vi "TestInfo.vi"(4 "Error In":errorcluster, 7 "Command":string) -> (0 "Error Out":errorcluster, 3 "Response":string)   [LabVIEW 2018]
uses:
  MOKO_LabViewLibrary/MokoLowLevel/MokoLowLovelControl/MLLC_Mode.ctl
  data/IZRCSM.ctl
panel:
  in  "Utility name":string="IZRCSM"
  in  "Error Code":i32=5475
  in  "Settings":T2
  in  "Mode":T3=enum."Check"
  # "TestInfo"
  # "Default Settings"
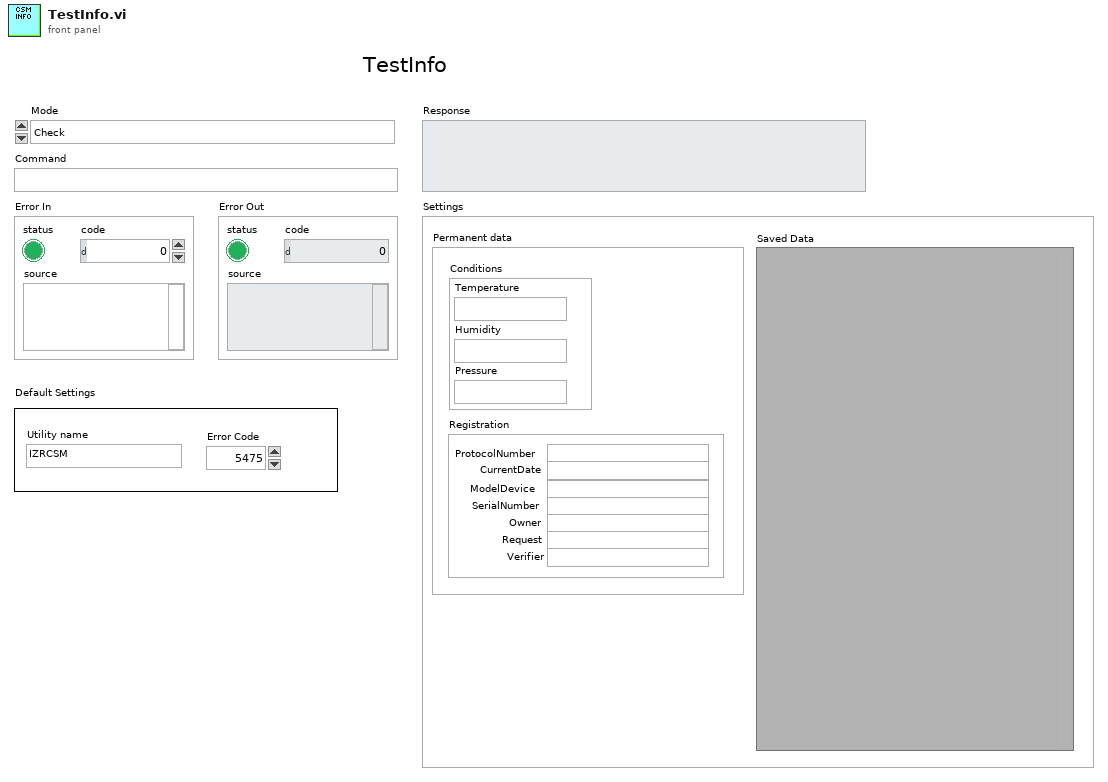
[diagram p1: front panel]
types:
  T1 = typedef "IZRCSM.ctl" = cluster{"Conditions":cluster{"Temperature":string, "Humidity":string, "Pressure":string}, "Registration":cluster{"ProtocolNumber":string, "CurrentDate":string, "ModelDevice":string, "SerialNumber":string, "Owner":string, "Request":string, "Verifier":string}}
  T2 = cluster{"Saved Data":variant, "Permanent data":T1}
  T3 = typedef "MLLC_Mode.ctl" = enum16{"get", "set", "close", "Init", "Check"}
  T4 = typedef "MLLC_Error.ctl" = errorcluster
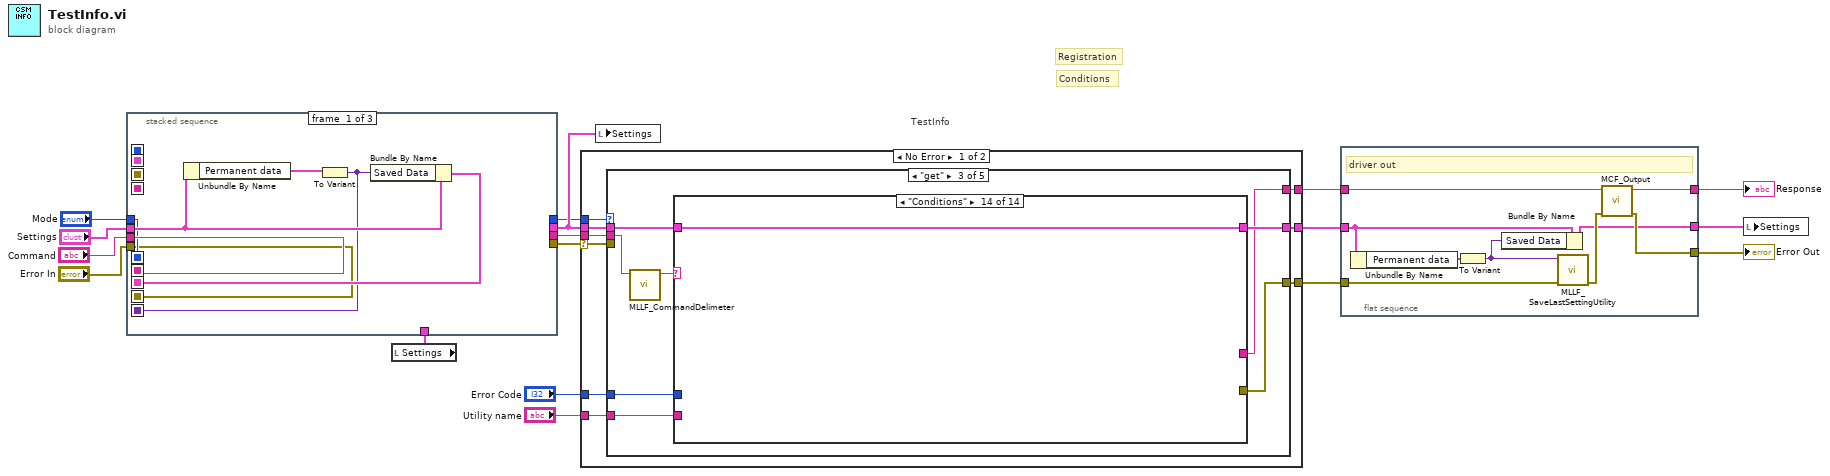
[diagram p0: block diagram]
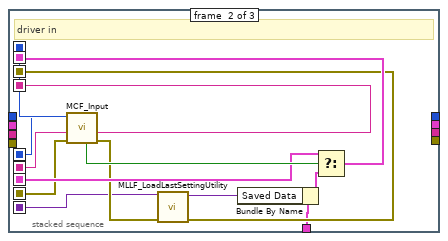
[diagram p2: hidden frame]
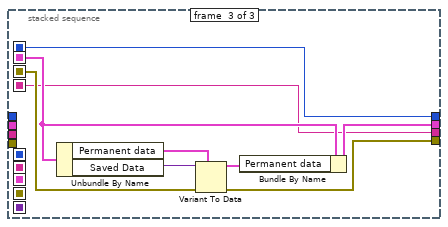
[diagram p3: hidden frame]
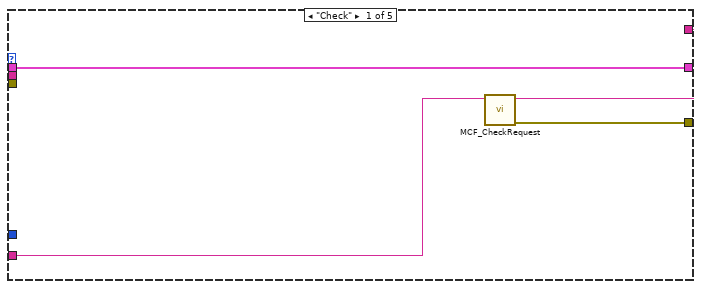
[diagram p4: hidden frame]
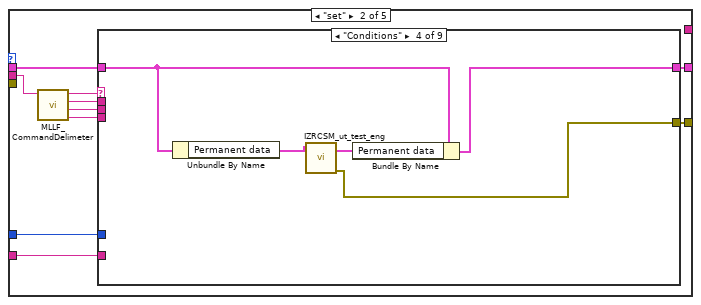
[diagram p5: hidden frame]
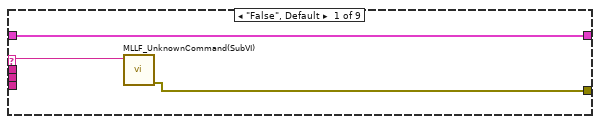
[diagram p6: hidden frame]
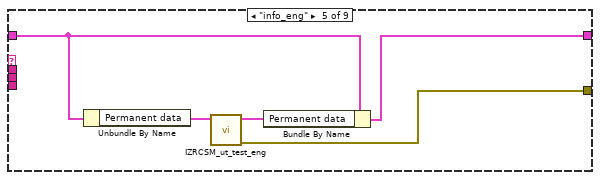
[diagram p9: hidden frame]
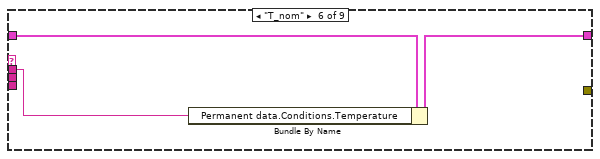
[diagram p10: hidden frame]
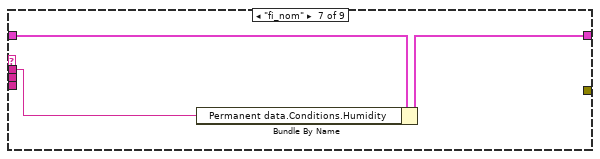
[diagram p11: hidden frame]
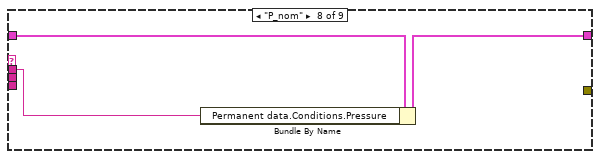
[diagram p12: hidden frame]
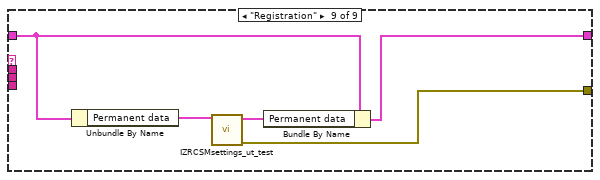
[diagram p13: hidden frame]
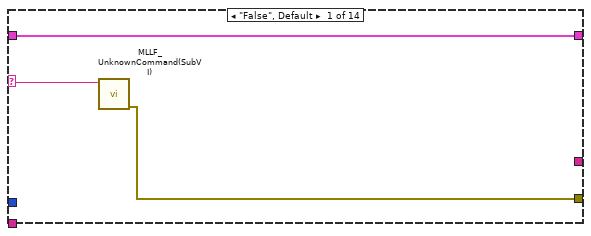
[diagram p14: hidden frame]
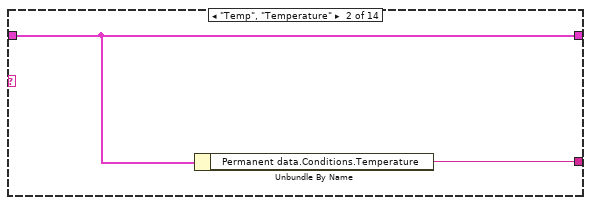
[diagram p15: hidden frame]
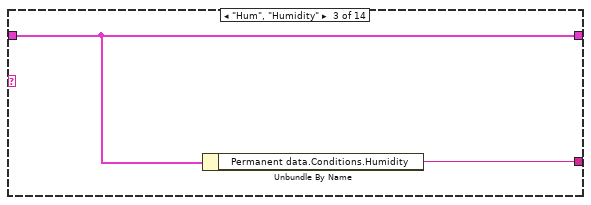
[diagram p16: hidden frame]
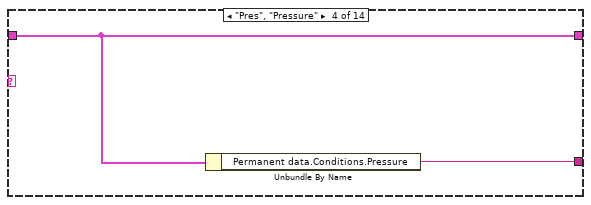
[diagram p17: hidden frame]
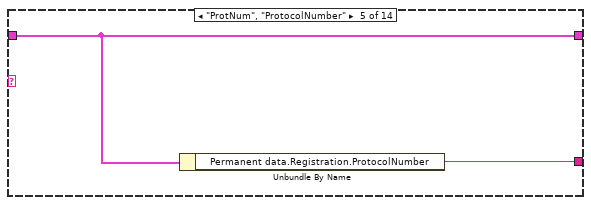
[diagram p18: hidden frame]
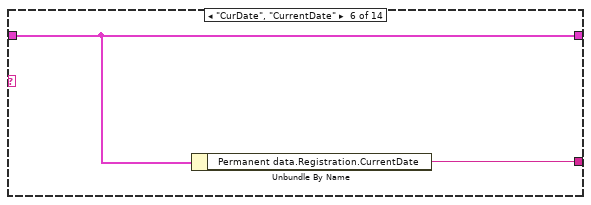
[diagram p19: hidden frame]
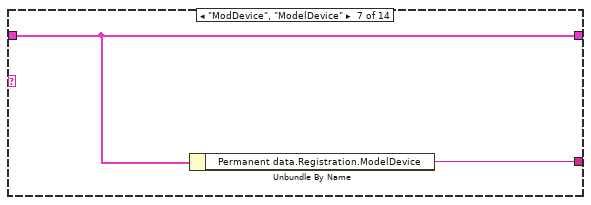
[diagram p20: hidden frame]
diagram:
  # "Conditions"
  # "Registration"
  # "TestInfo"
  n1 = local read "Settings"() -> (w12:T2)
  n2 = stacked-sequence {
    seq-local: [w20 _ _] -> [_ w36 _]
    seq-local: [w19 _ _] -> [_ w37 _]
    seq-local: [w22 _ _] -> [_ w32 _]
    seq-local: [w18 _ _] -> [_ w31 _]
    seq-local: [w21 _ _] -> [_ w26 _]
    seq-local: [_ w27 _] -> [_ _ w43]
    seq-local: [_ w38 _] -> [_ _ w40]
    seq-local: [_ w35 _] -> [_ _ w39]
    seq-local: [_ w34 _] -> [_ _ w44]
    tunnel: "Command" -> [w20 _ _]
    tunnel: "Mode" -> [w19 _ _]
    tunnel: "Error In" -> [w18 _ _]
    tunnel: "Settings" -> [w23 _ _]
    tunnel: w12 -> [_ w25 _]
    tunnel: [_ _ w39] -> w8
    tunnel: [_ _ w42] -> w11
    tunnel: [_ _ w41] -> w10
    tunnel: [_ _ w40] -> w9
    frame #0 {
      n3 = Unbundle By Name(w23) -> ("Permanent data"=w24:T1)
      n4 = To Variant(anything=w24) -> (Variant=w21:variant)
      n5 = Bundle By Name(cluster=w23, "Saved Data"=w21) -> (w22:T2)
    }
    frame #1 {
      # "driver in"
      n6 = call "MCF_Input.vi"("Error In"=w31, "Command in"=w36, "Mode in"=w37) -> ("Error Out"=w30:errorcluster, "Command out"=w35:string, "Mode out"=w38:T3, "Boolean"=w33:bool)  [unwired: 5 in]
      n7 = call "MLLF_LoadLastSettingUtility.vi"("Error In"=w30, "Save data in"=w26) -> ("Error Out"=w27:errorcluster, "Save data out"=w29:variant)  [unwired: 8 in]
      n8 = Bundle By Name(cluster=w25, "Saved Data"=w29) -> (w28:T2)
      n9 = Select(t=w32, s=w33, f=w28) -> (s? t:f=w34:T2)
    }
    frame #2 {
      n10 = Unbundle By Name(w44) -> ("Permanent data"=w45:T1, "Saved Data"=w47:variant)
      n11 = Variant To Data(error in=w43, type=w45, Variant=w47) -> (data=w46:T1, error out=w41:errorcluster)
      n12 = Bundle By Name(cluster=w44, "Permanent data"=w46) -> (w42:T2)
    }
  }
  n13 = case shown="No Error" w10 {
    selector: w10 -> [w52 w137]
    tunnel: [w54 w137] -> w16
    tunnel: w9 -> [w56 _]
    tunnel: [w55 _] -> w14
    tunnel: w8 -> [w53 _]
    tunnel: w11 -> [w49 w136]
    tunnel: "Error Code" -> [w51 _]
    tunnel: "Utility name" -> [w50 _]
    tunnel: [w48 w136] -> w15
    frame No Error {
      n14 = case shown="\"get\"" w56 {
        tunnel: [w58 _ w101 _ _] -> w55
        tunnel: [w57 w69 w100 _ _] -> w54
        tunnel: w53 -> [_ w70 w107 _ _]
        tunnel: w52 -> [_ _ _ _ _]
        tunnel: w51 -> [_ w68 w105 _ _]
        tunnel: w50 -> [w59 w65 w104 _ _]
        tunnel: w49 -> [w60 w67 w106 w134 w135]
        tunnel: [w60 w66 w103 w134 w135] -> w48
        frame "Check" {
          n15 = call "MCF_CheckRequest.vi"("Driver Name"=w59) -> ("Error Out"=w57:errorcluster, "Output String"=w58:string)  [unwired: 9 in]
        }
        frame "set" {
          n16 = call "MLLF_CommandDelimeter.vi"("command with param"=w70) -> ("param 3"=w61:string, "param 2"=w62:string, "param 1"=w63:string, "command"=w64:string)  [unwired: 6 in, 1 out]
          n17 = case shown="\"Conditions\"" w64 {
            selector: w64 -> [w72 _ _ _ _ _ _ _ _]
            tunnel: w63 -> [_ _ _ _ _ w86 w89 w92 _]
            tunnel: [w71 _ _ w76 w85 _ _ _ w99] -> w69
            tunnel: w68 -> [_ _ _ _ _ _ _ _ _]
            tunnel: w67 -> [w73 w74 w75 w80 w84 w88 w91 w94 w97]
            tunnel: [w73 w74 w75 w79 w83 w87 w90 w93 w98] -> w66
            tunnel: w65 -> [_ _ _ _ _ _ _ _ _]
            tunnel: w62 -> [_ _ _ _ _ _ _ _ _]
            tunnel: w61 -> [_ _ _ _ _ _ _ _ _]
            frame "False", Default {
              n18 = call "MLLF_UnknownCommand(SubVI).vi"("Unknown command"=w72) -> ("error out"=w71:errorcluster)  [unwired: 10 in]
            }
            frame "<----MAIN FUNCTIONS---->" {
            }
            frame "---------ADDITIONAL---------" {
            }
            frame "Conditions" {
              n19 = Unbundle By Name(w80) -> ("Permanent data"=w78:T1)
              n20 = call "IZRCSM_ut_test_eng.vi"("CSMinfo in"=w78) -> ("Error Out"=w76:errorcluster, "CSMinfo out"=w77:T1)  [unwired: 9 in]
              n21 = Bundle By Name(cluster=w80, "Permanent data"=w77) -> (w79:T2)
            }
            frame "info_eng" {
              n22 = Unbundle By Name(w84) -> ("Permanent data"=w81:T1)
              n23 = call "IZRCSM_ut_test_eng.vi"("CSMinfo in"=w81) -> ("Error Out"=w85:errorcluster, "CSMinfo out"=w82:T1)  [unwired: 9 in]
              n24 = Bundle By Name(cluster=w84, "Permanent data"=w82) -> (w83:T2)
            }
            frame "T_nom" {
              n25 = Bundle By Name(cluster=w88, "Permanent data.Conditions.Temperature"=w86) -> (w87:T2)
            }
            frame "fi_nom" {
              n26 = Bundle By Name(cluster=w91, "Permanent data.Conditions.Humidity"=w89) -> (w90:T2)
            }
            frame "P_nom" {
              n27 = Bundle By Name(cluster=w94, "Permanent data.Conditions.Pressure"=w92) -> (w93:T2)
            }
            frame "Registration" {
              n28 = Unbundle By Name(w97) -> ("Permanent data"=w96:T1)
              n29 = call "IZRCSMsettings_ut_test.vi"("CSMinfo in"=w96) -> ("Error Out"=w99:errorcluster, "CSMinfo out"=w95:T1)  [unwired: 9 in]
              n30 = Bundle By Name(cluster=w97, "Permanent data"=w95) -> (w98:T2)
            }
          }
        }
        frame "get" {
          n31 = call "MLLF_CommandDelimeter.vi"("command with param"=w107) -> ("command"=w102:string)  [unwired: 6 in, 4 out]
          n32 = case shown="\"Conditions\"" w102 {
            selector: w102 -> [w109 _ _ _ _ _ _ _ _ _ _ _ _ _]
            tunnel: [w108 _ _ _ _ _ _ _ _ _ _ _ _ _] -> w100
            tunnel: w105 -> [_ _ _ _ _ _ _ _ _ _ _ _ _ _]
            tunnel: [w110 w111 w113 w115 w117 w119 w121 w123 w125 w127 w129 w131 w132 w133] -> w103
            tunnel: w106 -> [w110 w111 w113 w115 w117 w119 w121 w123 w125 w127 w129 w131 w132 w133]
            tunnel: w104 -> [_ _ _ _ _ _ _ _ _ _ _ _ _ _]
            tunnel: [_ w112 w114 w116 w118 w120 w122 w124 w126 w128 w130 _ _ _] -> w101
            frame "False", Default {
              n33 = call "MLLF_UnknownCommand(SubVI).vi"("Unknown command"=w109) -> ("error out"=w108:errorcluster)  [unwired: 10 in]
            }
            frame "Temp", "Temperature" {
              n34 = Unbundle By Name(w111) -> ("Permanent data.Conditions.Temperature"=w112:string)
            }
            frame "Hum", "Humidity" {
              n35 = Unbundle By Name(w113) -> ("Permanent data.Conditions.Humidity"=w114:string)
            }
            frame "Pres", "Pressure" {
              n36 = Unbundle By Name(w115) -> ("Permanent data.Conditions.Pressure"=w116:string)
            }
            frame "ProtNum", "ProtocolNumber" {
              n37 = Unbundle By Name(w117) -> ("Permanent data.Registration.ProtocolNumber"=w118:string)
            }
            frame "CurDate", "CurrentDate" {
              n38 = Unbundle By Name(w119) -> ("Permanent data.Registration.CurrentDate"=w120:string)
            }
            frame "ModDevice", "ModelDevice" {
              n39 = Unbundle By Name(w121) -> ("Permanent data.Registration.ModelDevice"=w122:string)
            }
            frame "SerialNumber", "SerNumb" {
              n40 = Unbundle By Name(w123) -> ("Permanent data.Registration.SerialNumber"=w124:string)
            }
            frame "Owner" {
              n41 = Unbundle By Name(w125) -> ("Permanent data.Registration.Owner"=w126:string)
            }
            frame "Request" {
              n42 = Unbundle By Name(w127) -> ("Permanent data.Registration.Request"=w128:string)
            }
            frame "Verifier" {
              n43 = Unbundle By Name(w129) -> ("Permanent data.Registration.Verifier"=w130:string)
            }
            frame "_________________________________" {
            }
            frame "Registration" {
            }
            frame "Conditions" {
            }
          }
        }
        frame "close" {
        }
        frame "Init" {
        }
      }
    }
    frame Error {
    }
  }
  n44 = local write "Settings"(w11) -> ()
  n45 = flat-sequence {
    tunnel: [w146] -> w6
    tunnel: [w145] -> w4
    tunnel: w14 -> [w144]
    tunnel: w16 -> [w143]
    tunnel: w15 -> [w139]
    tunnel: [w141] -> w13
    frame #0 {
      # "driver out"
      n46 = Unbundle By Name(w139) -> ("Permanent data"=w138:T1)
      n47 = To Variant(anything=w138) -> (Variant=w140:variant)
      n48 = Bundle By Name(cluster=w139, "Saved Data"=w140) -> (w141:T2)
      n49 = call "MLLF_SaveLastSettingUtility.vi"("error in"=w143, "Saved Data"=w140) -> ("error out"=w142:T4)  [unwired: 8 in, 1 out]
      n50 = call "MCF_Output.vi"("Error In"=w142, "Input"=w144) -> ("Error Out"=w145:errorcluster, "Output"=w146:string)  [unwired: 8 in]
    }
  }
  n51 = local write "Settings"(w13) -> ()
  "Response" <- w6
  "Error Out" <- w4
